vi "Show_Trace_Database.vi"() -> ()   [LabVIEW 2016, in "data.citadel.lvclass"]
uses:
  data.citadel.lvclass
  <vilib>/lvdsc/historical/Read Trace (Numeric).vi
  <vilib>/lvdsc/NI_DSC.lvlib
panel:
  out "# stops":i32
  out "quality":dbl format="%.3f"
  out "historical trace":cluster{"timestamps":timestamp[], "data":dbl[]} {"data" format="%.6f"; "timestamps" format="%<%X\n%x>T"}
  out "output cluster":cluster{"timestamps":timestamp[], "data":dbl[]}
  out "System XY Graph":cluster{"timestamps":timestamp[], "data":dbl[]}(graph)
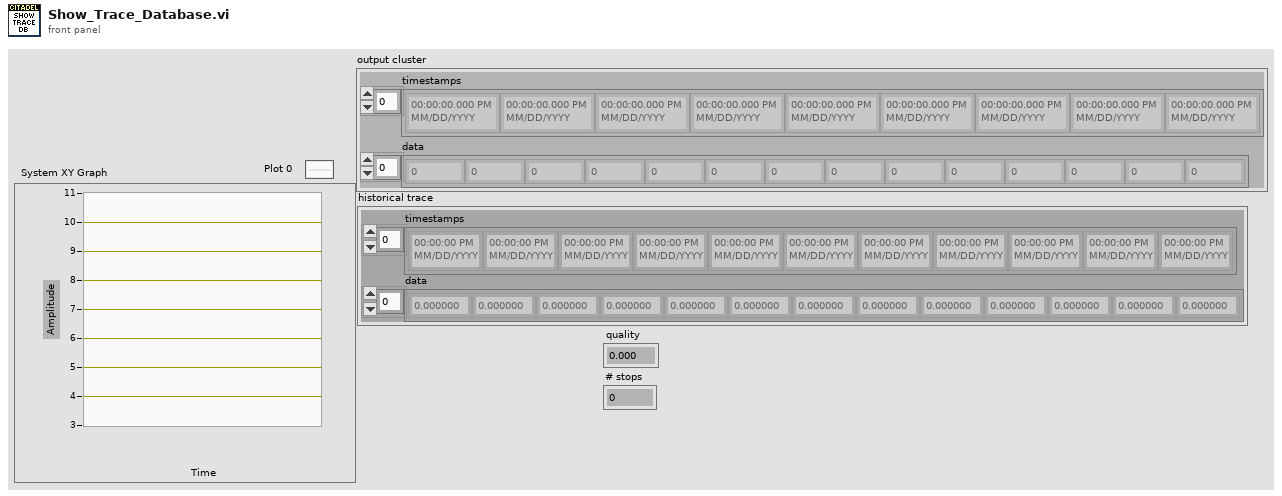
[diagram p1: front panel]
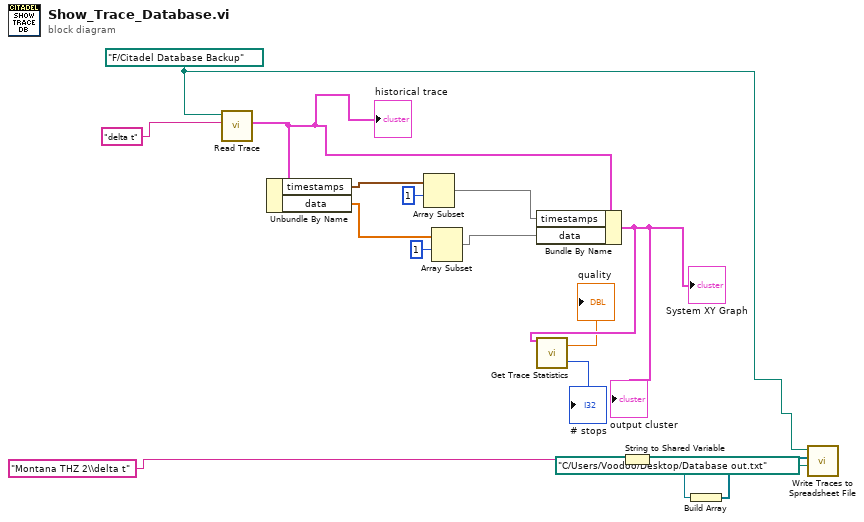
[diagram p0: block diagram]
diagram:
  w4 = path "F:/Citadel Database Backup" ("database URL")
  n1 = call-poly <vilib>:"Read Trace.vi"("trace name"="delta t" ("regular expression"), "database URL"=w4) -> ("historical trace"=w10:cluster{"timestamps":timestamp[], "data":dbl[]})  [unwired: 6 in, 3 out]
  "historical trace" <- w10
  n2 = Unbundle By Name(w10) -> ("timestamps"=w16:timestamp[], "data"=w15:dbl[])
  n3 = Array Subset(array=w16, index=1) -> (w14:timestamp[])  [unwired: 1 in]
  n4 = Array Subset(array=w15, index=1) -> (w13:dbl[])  [unwired: 1 in]
  n5 = Bundle By Name(cluster=w10, "timestamps"=w14, "data"=w13) -> (w9:cluster{"timestamps":timestamp[], "data":dbl[]})
  "System XY Graph" <- w9
  "output cluster" <- w9
  n6 = call <vilib>:"Get Trace Statistics.vi"("historical trace"=w9) -> ("quality"=→"quality":dbl, "# stops"=→"# stops":i32)  [unwired: 7 in, 6 out]
  n7 = String to Shared Variable(0:"Montana THZ 2\\delta t" ("regular expression")) -> (2:w3:refnum<k21>)  [unwired: 1 out]
  n8 = Build Array(w3) -> (w2:refnum<k21>[])
  n9 = call <vilib>:"Write Traces to Spreadsheet File.vi"("output file path"=path "C:/Users/Voodoo/Desktop/Database out.txt", "trace names"=w2, "database URL"=w4) -> ()  [unwired: 6 in, 3 out]
